vi "Adjust Dashboard Window.vi"(6 "Sizing Refnums":T1, 9 "Size Constraints":cluster{"min tab width":i32, "w/h":dbl}, 10 "VI":refnum<vi>, 11 "WIn Mode":refnum<notifier>) -> ()   [LabVIEW 2016]
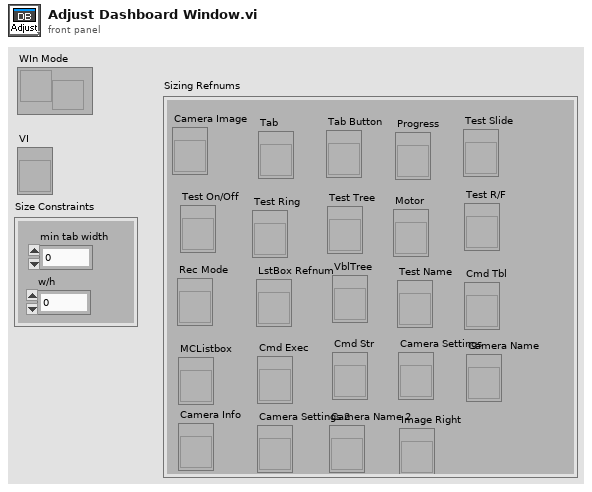
[diagram p1: front panel]
types:
  T1 = cluster{"Camera Image":refnum<vi>, "Tab":refnum<vi>, "Tab Button":refnum<vi>, "Rec Mode":refnum<vi>, "Test Slide":refnum<vi>, "Test On/Off":refnum<vi>, "Test Ring":refnum<vi>, "Test R/F":refnum<vi>, "Test Name":refnum<vi>, "Motor":refnum<vi>, "Progress":refnum<vi>, "LstBox Refnum":refnum<vi>, "Test Tree":refnum<vi>, "VblTree":refnum<vi>, "Cmd Tbl":refnum<vi>, "MCListbox":refnum<vi>, "Cmd Exec":refnum<vi>, "Cmd Str":refnum<vi>, "Camera Settings":refnum<vi>, "Camera Name":refnum<vi>, "Camera Info":refnum<vi>, "Camera Settings 2":refnum<vi>, "Camera Name 2":refnum<vi>, "Image Right":refnum<vi>}
  T2 = typedef "LVRectTypeDef.ctl" = cluster{"Left":i16, "Top":i16, "Right":i16, "Bottom":i16}
  T3 = typedef "LVPointTypeDef.ctl" = cluster{"Horizontal":i16, "Vertical":i16}
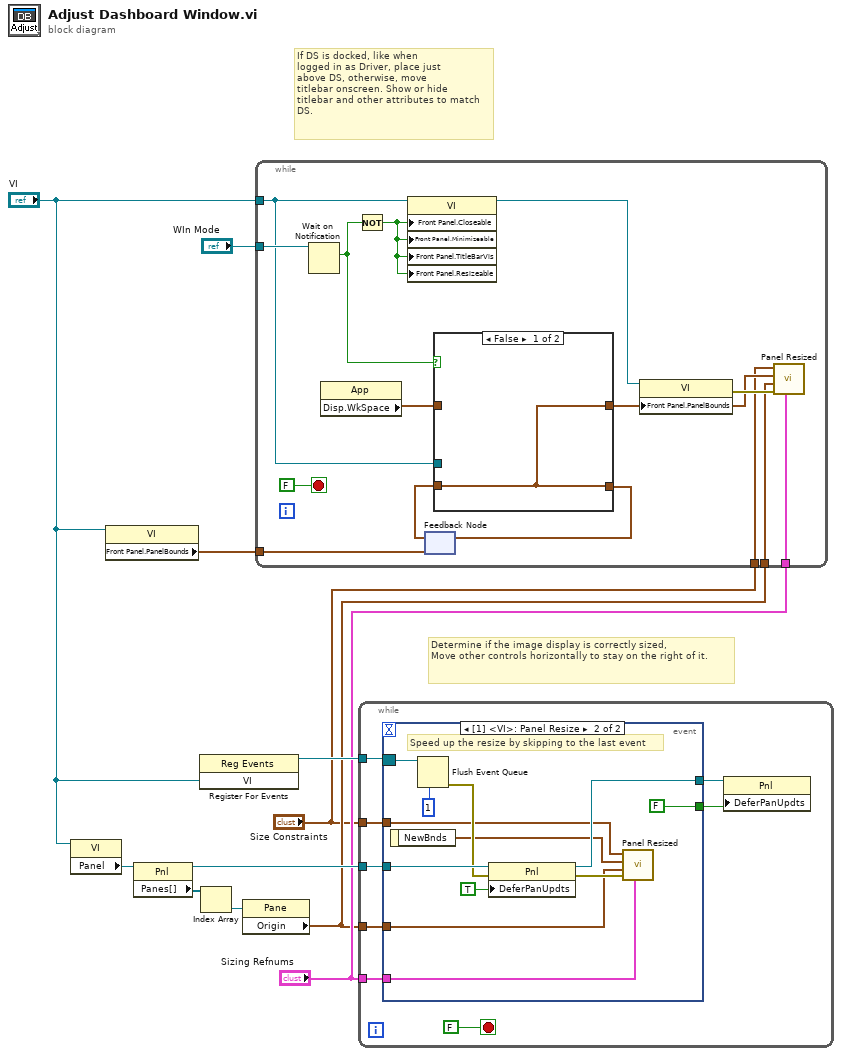
[diagram p0: block diagram]
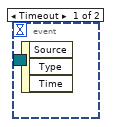
[diagram p2: hidden frame]
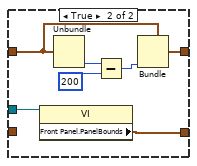
[diagram p3: hidden frame]
diagram:
  # "Determine if the image display is correctly sized,\nMove other controls horizontally to stay on the right of it."
  # "If DS is docked, like when\nlogged in as Driver, place just\nabove DS, otherwise, move\ntitlebar onscreen. Show or hide\ntitlebar and other attributes to match\nDS."
  n1 = property class="VI"(reference="VI") -> ("Panel"=w9:refnum<vi>)  [unwired: 1 in, 2 out]
  n2 = property class="VI"(reference="VI") -> ("Front Panel.PanelBounds"=w2:T2)  [unwired: 1 in, 2 out]
  n3 = property class="Pnl"(reference=w9) -> (reference out=w6:refnum<vi>, "Panes[]"=w8:refnum<vi>[])  [unwired: 1 in, 1 out]
  n4 = register-events("VI") -> (reference out=w10:refnum<event-registration>)  [unwired: 2 in, 1 out]
  n5 = Index Array(array=w8) -> (element=w7:refnum<vi>)  [unwired: 1 in]
  n6 = property class="Pane"(reference=w7) -> ("Origin"=w4:T3)  [unwired: 1 in, 2 out]
  n7 = while {
    tunnel: "WIn Mode" -> [w25]
    tunnel: "VI" -> [w16]
    tunnel: "Sizing Refnums" -> [w21]
    tunnel: w4 -> [w20]
    tunnel: "Size Constraints" -> [w18]
    tunnel: w2 -> [w13]
    stop <- FALSE stop-if-true
    n8 = Wait on Notification(notifier=w25) -> (notification=w17:bool)  [unwired: 3 in, 3 out]
    n9 = property class="App"() -> ("Disp.WkSpace"=w24:T2)  [unwired: 2 in, 2 out]
    n10 = Not(x=w17) -> (.not. x?=w12:bool)
    n11 = property class="VI"(reference=w16, "Front Panel.Closeable"=w12, "Front Panel.Minimizeable"=w12, "Front Panel.TitleBarVis"=w12, "Front Panel.Resizeable"=w12) -> (reference out=w23:refnum<vi>)  [unwired: 1 in, 1 out]
    n12 = feedback #1(w13) -> (w14:T2)
    n13 = case shown="False" w17 {
      tunnel: w24 -> [_ w30]
      tunnel: [w27 w31] -> w19
      tunnel: w16 -> [_ w29]
      tunnel: [w27 w28] -> w15
      tunnel: w14 -> [w27 _]
      frame False {
      }
      frame True {
        n14 = property class="VI"(reference=w29) -> ("Front Panel.PanelBounds"=w28:T2)  [unwired: 1 in, 2 out]
        n15 = Unbundle(w30) -> ("Bottom"=w34:i16)  [unwired: 3 out]
        n16 = Subtract(x=w34, y=200) -> (x-y=w32:i32)
        n17 = Bundle(cluster=w30, "Bottom"=w32) -> (w31:T2)  [unwired: 3 out]
      }
    }
    n18 = feedback-in #1(w15) -> ()
    n19 = property class="VI"(reference=w23, "Front Panel.PanelBounds"=w19) -> (error out=w22:errorcluster)  [unwired: 1 in, 1 out]
    n20 = call "Panel Resized.vi"("Sizing Refnums"=w21, "error in (no error)"=w22, "Origin"=w20, "NewBnds"=w19, "Size Constraints"=w18) -> ()  [unwired: 6 in, 1 out]
  }
  n21 = while {
    tunnel: w10 -> [w41]
    tunnel: "Sizing Refnums" -> [w40]
    tunnel: "Size Constraints" -> [w39]
    tunnel: w4 -> [w38]
    tunnel: w6 -> [w37]
    stop <- FALSE stop-if-true
    n22 = event shown="[1] <VI>: Panel Resize" {
      selector: w41 -> [_ w51]
      dyn-events: _ -> [_ _]
      timeout: _ -> [_ _]
      tunnel: w40 -> [_ w43]
      tunnel: w39 -> [_ w46]
      tunnel: w38 -> [_ w44]
      tunnel: w37 -> [_ w54]
      tunnel: [_ FALSE ("Defer Panel Updates")] -> w36
      tunnel: [_ w48] -> w35
      event Timeout {
        n23 = event-data() -> ()  [unwired: 1 in, 3 out]
      }
      event Panel Resize {
        # "Speed up the resize by skipping to the last event"
        n24 = event-data() -> ("NewBnds"=w45:T2)  [unwired: 1 in]
        n25 = Flush Event Queue(0:w51, 5:1 ("keep most recent")) -> (11:w49:errorcluster)  [unwired: 4 in, 2 out]
        n26 = property class="Pnl"(reference=w54, error in=w49, "DeferPanUpdts"=TRUE ("Defer Panel Updates")) -> (reference out=w48:refnum<vi>, error out=w47:errorcluster)
        n27 = call "Panel Resized.vi"("Sizing Refnums"=w43, "error in (no error)"=w47, "Origin"=w44, "NewBnds"=w45, "Size Constraints"=w46) -> ()  [unwired: 6 in, 1 out]
      }
    }
    n28 = property class="Pnl"(reference=w35, "DeferPanUpdts"=w36) -> ()  [unwired: 1 in, 2 out]
  }
